vi "svfa_Average Array with Avg Checks (real) (1 Ch).vi"(0 "spectrum":dbl[](array[numeric]) format="%.2f", 1 "processing control":T1(ring), 7 "averaging parameters":T2={"averaging mode"=enum."No averaging", "weighting mode"=enum."Linear", "number of averages"=10, "linear mode"=enum."Auto restart"}, 11 "error in (no error)":errorcluster) -> (4 "average spectrum":dbl[](array[numeric]) format="%.2f", 6 "new spectrum ready":bool, 8 "averaging done":bool, 10 "averages completed":dbl, 15 "error out":errorcluster)   [LabVIEW 2017]
uses:
  <vilib>/addons/_NISVFA/_Shared subVIs/Spectrum Averaging/svfa_Average Array (real) No State.vi
  <vilib>/addons/_NISVFA/_Shared subVIs/Spectrum Averaging/svfa_No Average Array (real).vi
  <vilib>/addons/_NISVFA/_Shared subVIs/Spectrum Averaging/svfa_Average Array (real).vi
  <vilib>/addons/_NISVFA/_Shared subVIs/Spectrum Averaging/svfa_Peak Hold Array.vi
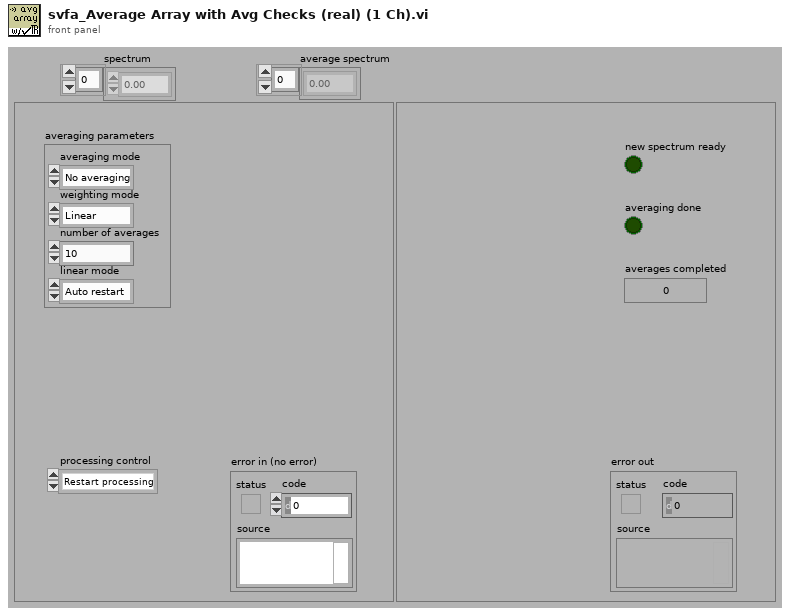
[diagram p1: front panel]
types:
  T1 = enum16{"Restart processing", "Continue processing", "Skip processing"}
  T2 = cluster{"averaging mode":enum16{"No averaging", "Vector averaging", "RMS averaging", "Peak hold"}, "weighting mode":enum16{"Linear", "Exponential"}, "number of averages":u32, "linear mode":enum16{"One shot", "Auto restart"}}
  T3 = cluster{"complex FFT":cdb[], "real FFT":dbl[], "f0":dbl, "df":dbl, "averages completed":dbl, "averaging parameters":cluster{"averaging mode":enum16{"No averaging", "Vector averaging", "RMS averaging", "Peak hold"}, "weighting mode":enum16{"Linear", "Exponential"}, "number of averages":u32, "linear mode":enum16{"One shot", "Auto restart"}}}
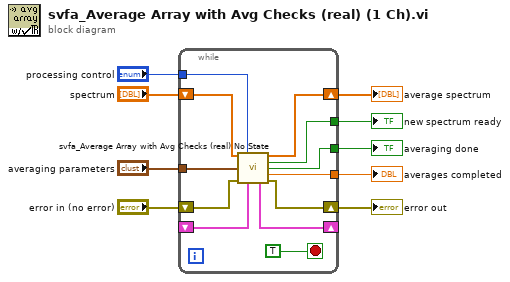
[diagram p0: block diagram]
diagram:
  n1 = while {
    tunnel: "processing control" -> [w14]
    shift-left: _ -> [w15]
    shift-right: [w16] -> _
    tunnel: [w10] -> w4
    tunnel: [w18] -> w5
    tunnel: [w19] -> w6
    tunnel: "averaging parameters" -> [w13]
    shift-right: [w20] -> w7
    shift-left: "spectrum" -> [w21]
    shift-right: [w11] -> w3
    shift-left: "error in (no error)" -> [w12]
    stop <- TRUE stop-if-true
    n2 = call <vilib>:"svfa_Average Array with Avg Checks (real) No State.vi"("spectrum"=w21, "processing control"=w14, "averaging parameters"=w13, "error in"=w12, "averaging state info"=w15) -> ("avg spectrum"=w20:dbl[], "new spectrum ready"=w19:bool, "averaging done"=w18:bool, "averages completed"=w10:dbl, "averaging state info"=w16:T3, "error out"=w11:errorcluster)  [unwired: 5 in]
  }
  "average spectrum" <- w7
  "averages completed" <- w4
  "new spectrum ready" <- w6
  "averaging done" <- w5
  "error out" <- w3
